vi "RemoveCamerasFromActiveList.vi"(8 "error in (no error)":errorcluster, 10 "camera to remove":string, 11 "config":T2) -> (0 "error out":errorcluster, 2 "cameras removed":T1[](array[typedef]), 3 "config out":T2)   [LabVIEW 2017, in "IrManageCameras.lvlib"]
uses:
  <vilib>/addons/InsightCM/Devices/Shared/Ir/IrManageCameras/IrManageCameras.lvlib
  <vilib>/addons/InsightCM/Devices/Shared/Ir/IrManageCameras/controls/config.ctl
  <vilib>/addons/InsightCM/Devices/Shared/Ir/IrManageCameras/controls/camera.ctl
  InsightCM/Devices/WebServices/Ir/DataAccessors/action.ctl
  InsightCM/Devices/WebServices/Ir/DataAccessors/VisionWebServiceData.lvlib
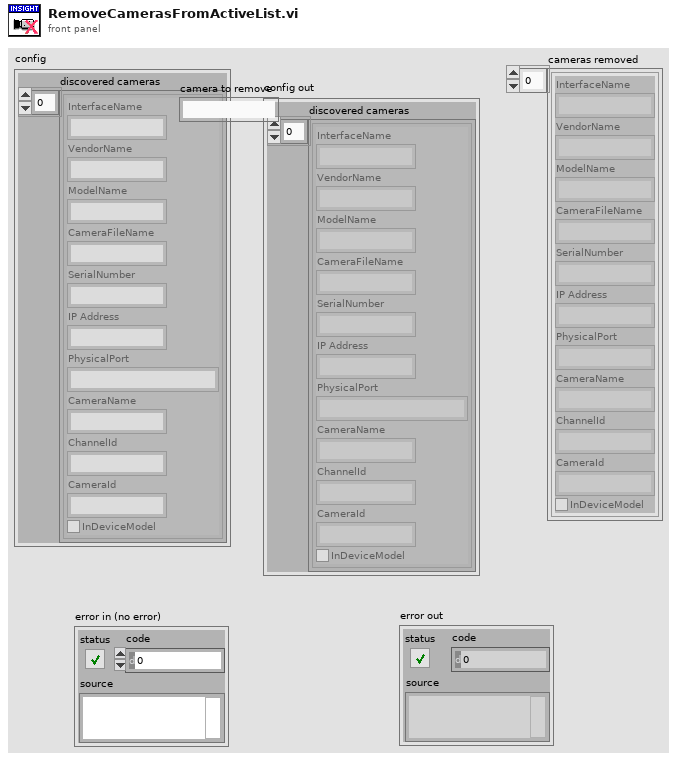
[diagram p1: front panel]
types:
  T1 = typedef "IrManageCameras.lvlib/camera.ctl" = cluster{"InterfaceName":string, "VendorName":string, "ModelName":string, "CameraFileName":string, "SerialNumber":string, "IP Address":string, "PhysicalPort":string, "CameraName":string, "ChannelId":string, "CameraId":string, "InDeviceModel":bool}
  T2 = typedef "IrManageCameras.lvlib/config.ctl" = cluster{"discovered cameras":T1[]}
  T3 = typedef "VisionWebServiceData.lvlib/action.ctl" = enum16{"Get", "Set"}
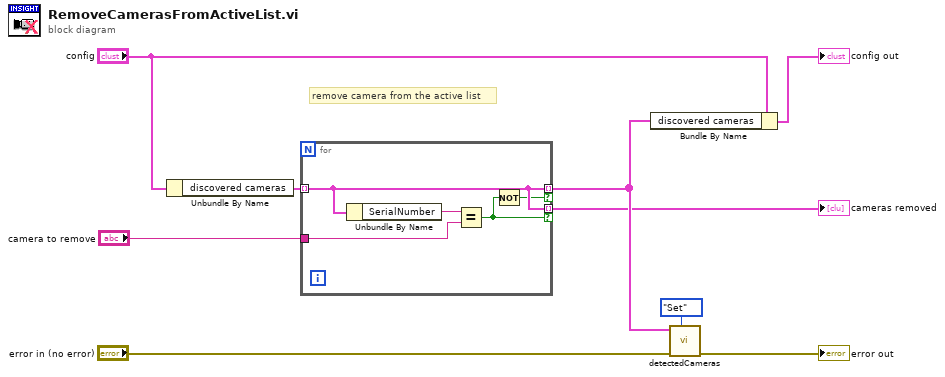
[diagram p0: block diagram]
diagram:
  # "remove camera from the active list"
  n1 = Unbundle By Name("config") -> ("discovered cameras"=w9:T1[])
  n2 = for {
    tunnel: w9 -> [w12] mode=indexing
    tunnel: "camera to remove" -> [w13]
    tunnel: [w12] -> w5 mode=indexing if=w10
    tunnel: [w12] -> w2 mode=indexing if=w11
    n3 = Unbundle By Name(w12) -> ("SerialNumber"=w14:string)
    n4 = Equal?(x=w14, y=w13) -> (x = y?=w11:bool)
    n5 = Not(x=w11) -> (.not. x?=w10:bool)
  }
  "cameras removed" <- w2
  n6 = Bundle By Name(cluster="config", "discovered cameras"=w5) -> (→"config out":T2)
  n7 = call "detectedCameras.vi"("action"=action."Set", "error in (no error)"="error in (no error)", "Discovered Cameras"=w5) -> ("error out"=→"error out":errorcluster)  [unwired: 7 in, 1 out]
